vi "Index2D.vi"(2 "Size":i32, 3 "Step":dbl) -> (0 "Y":dbl[][](array[numeric]), 1 "X":dbl[][](array[numeric]))   [LabVIEW 2009]
uses:
  <vilib>/Analysis/NI_AALBase.lvlib
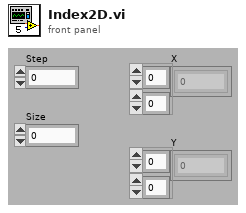
[diagram p1: front panel]
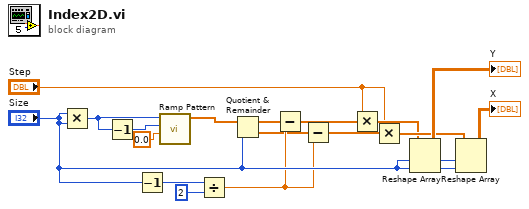
[diagram p0: block diagram]
diagram:
  n1 = Multiply(x="Size", y="Size") -> (x*y=w3:i32)
  n2 = Decrement(x=w3) -> (x-1=w2:i32)
  n3 = Decrement(x="Size") -> (x-1=w15:i32)
  n4 = call <vilib>:"Ramp Pattern.vi"("start"=0.0, "end"=w2, "samples"=w3) -> ("Ramp Pattern"=w4:dbl[])  [unwired: 7 in, 1 out]
  n5 = Divide(x=w15, y=2) -> (x/y=w8:dbl)
  n6 = Quotient & Remainder(x=w4, y="Size") -> (x-y*floor(x/y)=w5:dbl[], floor(x/y)=w7:dbl[])
  n7 = Subtract(x=w5, y=w8) -> (x-y=w9:dbl[])
  n8 = Subtract(x=w7, y=w8) -> (x-y=w10:dbl[])
  n9 = Multiply(x="Step", y=w9) -> (x*y=w12:dbl[])
  n10 = Multiply(x=w10, y="Step") -> (x*y=w13:dbl[])
  n11 = Reshape Array(w12, "Size", "Size") -> (→"Y":dbl[][])
  n12 = Reshape Array(w13, "Size", "Size") -> (→"X":dbl[][])
